vi "Alicat setpoint.vi"(2 "Setpoint":dbl format="%_4g", 3 "Unit ID":string="P", 4 "ALICAT COM Port":refnum<visa-resource-name>="COM5") -> ()   [LabVIEW 2023]
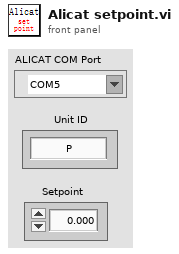
[diagram p1: front panel]
types:
  T1 = enum8{"2400", "9600", "19200", "38400", "57600", "115200", "Unknown"}
  T2 = cluster{"Unit ID":string, "Baud Rate":enum8{"2400", "9600", "19200", "38400", "57600", "115200", "Unknown"}, "ALICAT COM Port":refnum<visa-resource-name>}
  T3 = cluster{"Controller Full Scale":dbl, "Controller Select":u16, "Control Range":enum16{"Normal", "Inverted", "Bidirectional", "Unknown"}}
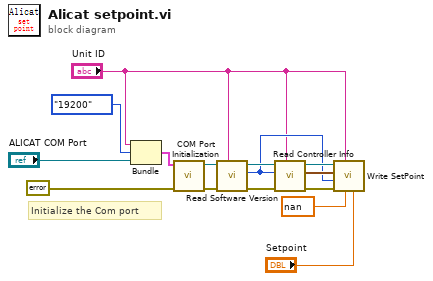
[diagram p0: block diagram]
diagram:
  # "Initialize the Com port"
  n1 = Bundle("Unit ID"="Unit ID", "Baud Rate"=T1."19200", "ALICAT COM Port"="ALICAT COM Port") -> (w2:T2)  [unwired: 1 in]
  n2 = call "COM Port Initialization.vi"("error in (no error)"=errorcluster {"status"=FALSE, "code"=0, "source"=""}, "Communication Settings"=w2) -> ("error out"=w15:errorcluster, "VISA Session Out"=w14:refnum<visa-resource-name>)  [unwired: 8 in]
  n3 = call "Read Software Version.vi"("Unit ID (A)"="Unit ID", "error in"=w15, "VISA Session In"=w14) -> ("error out"=w12:errorcluster, "Software Version"=w7:u8, "VISA Session Out"=w11:refnum<visa-resource-name>)  [unwired: 6 in]
  n4 = call "Read Controller Info.vi"("Unit ID (A)"="Unit ID", "error in"=w12, "Software Version"=w7, "VISA Session In"=w11) -> ("error out"=w10:errorcluster, "Controller Info out"=w9:T3, "VISA Session Out"=w8:refnum<visa-resource-name>)  [unwired: 4 in, 1 out]
  n5 = call "Write SetPoint.vi"("Setpoint"="Setpoint", "Previous Setpoint"=nan, "Unit ID (A)"="Unit ID", "error in"=w10, "Software Version"=w7, "Controller Info out"=w9, "VISA Session In"=w8) -> ()  [unwired: 1 in, 4 out]
